vi "sine_to_analog_output_configured.vi"() -> ()   [LabVIEW 2011]
uses:
  <vilib>/Utility/error.llb/DialogType.ctl
  <vilib>/DAQmx/write.llb/DAQmx Write (Analog 1D Wfm NChan NSamp).vi
  <vilib>/DAQmx/create/channels.llb/DAQmx Create Channel (AO-Voltage-Basic).vi
  <vilib>/DAQmx/configure/timing.llb/DAQmx Timing (Use Waveform).vi
  <vilib>/DAQmx/miscellaneous.llb/DAQmx Fill In Error Info.vi
  Program Files (x86)/National Instruments/LabVIEW 2011/resource/objmgr/daqmx.rc
panel:
  out "Resulting Frequency":dbl format="%.2f"
  out "Output Waveform":waveform(dbl)[](graph)
  in  "stop":bool
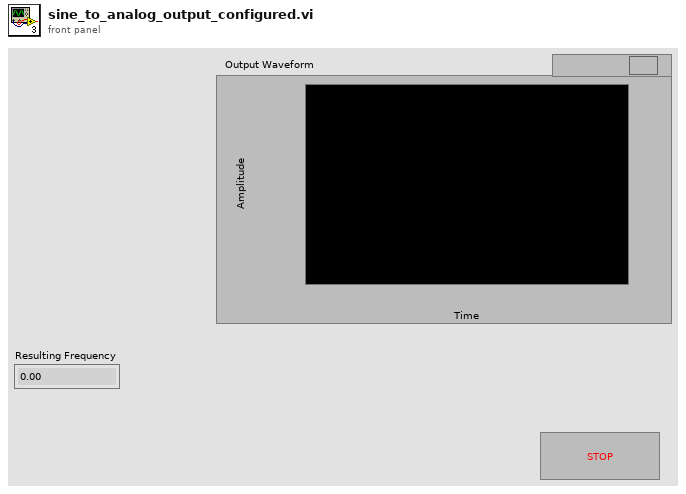
[diagram p1: front panel]
types:
  T1 = enum16{"Sine Wave", "Triangle Wave", "Square Wave", "Sawtooth Wave"}
  T2 = typedef "DialogType.ctl" = u16
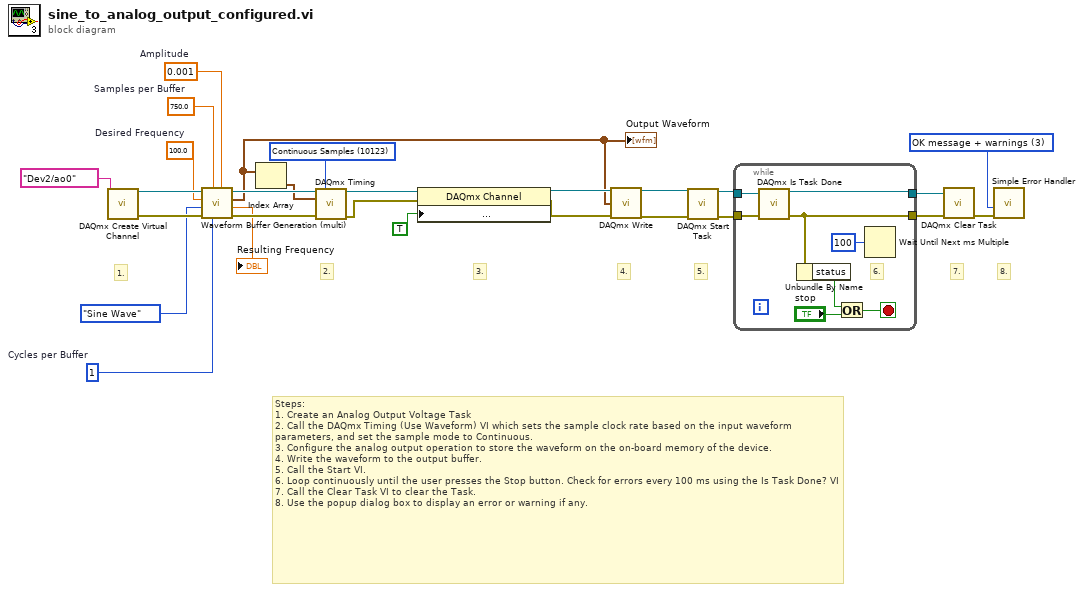
[diagram p0: block diagram]
diagram:
  w9 = 750.0  # Samples per Buffer
  w7 = 1  # Cycles per Buffer
  w1 = 0.001  # Amplitude
  w2 = 100.0  # Desired Frequency
  w17 = T2 3 items=["no dialog", "OK message", "continue or stop message", "OK message + warnings", "continue/stop + warnings"] ("type of dialog (OK msg:1)")
  w26 = 10123 items=["Finite Samples"=10178, "Continuous Samples"=10123] ("sample mode")
  # "7."
  # "8."
  # "5."
  # "Steps: \n1. Create an Analog Output Voltage Task\n2. Call the DAQmx Timing (Use Waveform) VI which sets the sample clock rate based on the input waveform parameters, and set the sample mode to Continuous.\n3. Configure the analog output operation to store the waveform on the on-board memory of the device.\n4. Write the waveform to the output buffer.\n5. Call the Start VI.\n6. Loop continuously until the user presses the Stop button. Check for errors every 100 ms using the Is Task Done? VI\n7. Call the Clear Task VI to clear the Task.\n8. Use the popup dialog box to display an error or warning if any."
  # "4."
  # "3."
  # "2."
  # "1."
  n1 = call-poly <vilib>:"DAQmx Create Virtual Channel.vi"("physical channels"=tag "Dev2/ao0") -> ("task out"=w11:refnum<k21>, "error out"=w13:errorcluster)  [unwired: 13 in]
  n2 = call "Waveform Buffer Generation (multi).vi"("Amplitude"=w1, "Cycles per Buffer"=w7, "Samples per Buffer"=w9, "error in (no error)"=w13, "Waveform Type"=T1."Sine Wave", "Desired Frequency"=w2, "task/channels in"=w11) -> ("error out"=w12:errorcluster, "Resulting Frequency"=→"Resulting Frequency":dbl, "Waveform"=w5:waveform(dbl)[], "task out"=w10:refnum<k21>)  [unwired: 1 out]
  "Output Waveform" <- w5
  n3 = Index Array(array=w5) -> (element=w4:waveform(dbl))  [unwired: 1 in]
  n4 = call-poly <vilib>:"DAQmx Timing.vi"("task/channels in"=w10, "sample mode"=w26, "waveform"=w4, "error in"=w12) -> ("task out"=w21:refnum<k21>, "error out"=w20:errorcluster)  [unwired: 10 in]
  n5 = property class="DAQmx Channel"(reference=w21, error in=w20, "Analog Output:General Properties:Advanced:Data Transfer and Memory:Use Only Onboard Memory"=TRUE ("AO.UseOnlyOnBrdMem")) -> (reference out=w19:refnum<k21>, error out=w18:errorcluster)
  n6 = call-poly <vilib>:"DAQmx Write.vi"("task/channels in"=w19, "data"=w5, "error in"=w18) -> ("task out"=w23:refnum<k21>, "error out"=w25:errorcluster)  [unwired: 10 in, 1 out]
  n7 = call <vilib>:"DAQmx Start Task.vi"("task/channels in"=w23, "error in"=w25) -> ("task out"=w27:refnum<k21>, "error out"=w24:errorcluster)  [unwired: 12 in]
  n8 = while {
    tunnel: w27 -> [w31]
    tunnel: [w29] -> w15
    tunnel: w24 -> [w30]
    tunnel: [w28] -> w14
    stop <- w35 stop-if-true
    # "6."
    n9 = call <vilib>:"DAQmx Is Task Done.vi"("task/channels in"=w31, "error in"=w30) -> ("task out"=w29:refnum<k21>, "error out"=w28:errorcluster)  [unwired: 11 in, 1 out]
    n10 = Unbundle By Name(w28) -> ("status"=w33:bool)
    n11 = Or(x=w33, y="stop") -> (x .or. y?=w35:bool)
    n12 = Wait Until Next ms Multiple(millisecond multiple=u32 100) -> ()  [unwired: 1 out]
  }
  n13 = call <vilib>:"DAQmx Clear Task.vi"("task in"=w15, "error in"=w14) -> ("error out"=w16:errorcluster)  [unwired: 13 in]
  n14 = call <vilib>:"Simple Error Handler.vi"("type of dialog (OK msg:1)"=w17, "error in (no error)"=w16) -> ()  [unwired: 3 in, 5 out]
